vi "Wrap Text.vi"(5 "Enabled? (T)":bool=TRUE, 7 "Formatting":T1="h2", 8 "Error in":errorcluster caption="Error in (no error)", 11 "String":string) -> (0 "Error out":errorcluster, 3 "Wrapped String":string)   [LabVIEW 2023, in "Confluence Formatting.lvlib"]
uses:
  Confluence Formatting.lvlib
  Types/Format Combo Box.ctl
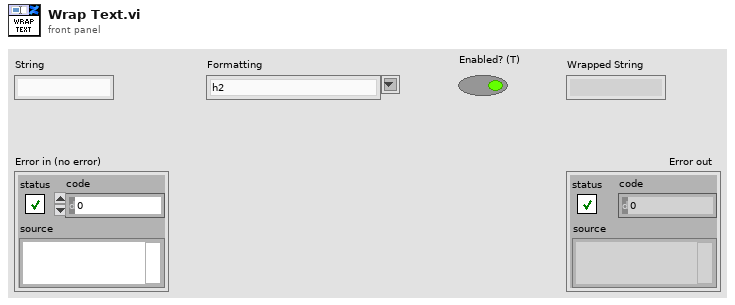
[diagram p1: front panel]
types:
  T1 = typedef "Confluence Formatting.lvlib/Format Combo Box.ctl" = string
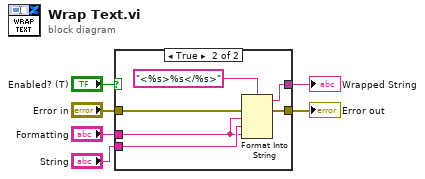
[diagram p0: block diagram]
diagram:
  n1 = case shown="True" "Enabled? (T)" {
    tunnel: "String" -> [_ w12]
    tunnel: "Formatting" -> [_ w11]
    tunnel: [_ w10] -> w4
    tunnel: "Error in" -> [w7 w9]
    tunnel: [w7 w8] -> w2
    frame False {
    }
    frame True {
      n2 = Format Into String(format string="<%s>%s</%s>", error in=w9, w11, w12, w11) -> (resulting string=w10:string, error out=w8:errorcluster)  [unwired: 1 in]
    }
  }
  "Wrapped String" <- w4
  "Error out" <- w2
